vi "swingup_accel_to_voltage.vi"(1 "theta_dot (rad/s)":dbl, 2 "u (m/s^2)":dbl, 3 "Rm (ohms)":dbl, 4 "Kt (N.m/A)":dbl, 5 "r (m)":dbl, 6 "m_arm (kg)":dbl) -> (0 "Vm (V)":dbl)   [LabVIEW 2010]
doc: "This VI calculates the motor voltage needed to achieve the desired pendulum pivot acceleration given."
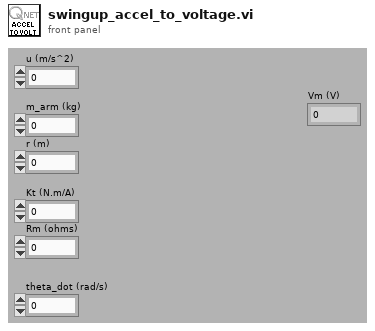
[diagram p1: front panel]
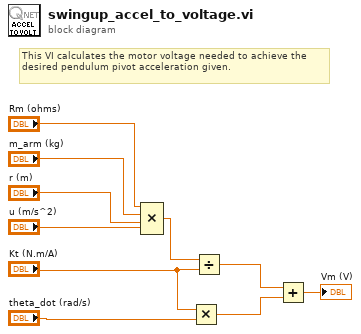
[diagram p0: block diagram]
diagram:
  # "This VI calculates the motor voltage needed to achieve the desired pendulum pivot acceleration given."
  n1 = Compound Arithmetic op=MULTIPLY("Rm (ohms)", "m_arm (kg)", "r (m)", "u (m/s^2)") -> (w10:dbl)
  n2 = Multiply(x="Kt (N.m/A)", y="theta_dot (rad/s)") -> (x*y=w8:dbl)
  n3 = Divide(x=w10, y="Kt (N.m/A)") -> (x/y=w9:dbl)
  n4 = Add(x=w9, y=w8) -> (x+y=→"Vm (V)":dbl)
